vi "Fixed width File Parser.vi"(9 "Length of Column":i32[](array[numeric]), 10 "Start Index":i32[](array[numeric]), 11 "Folder to Check":path) -> (3 "Parsed Data":string[][](array[string]))   [LabVIEW 2009]
uses:
  <vilib>/Utility/file.llb/Read From Spreadsheet File (string).vi
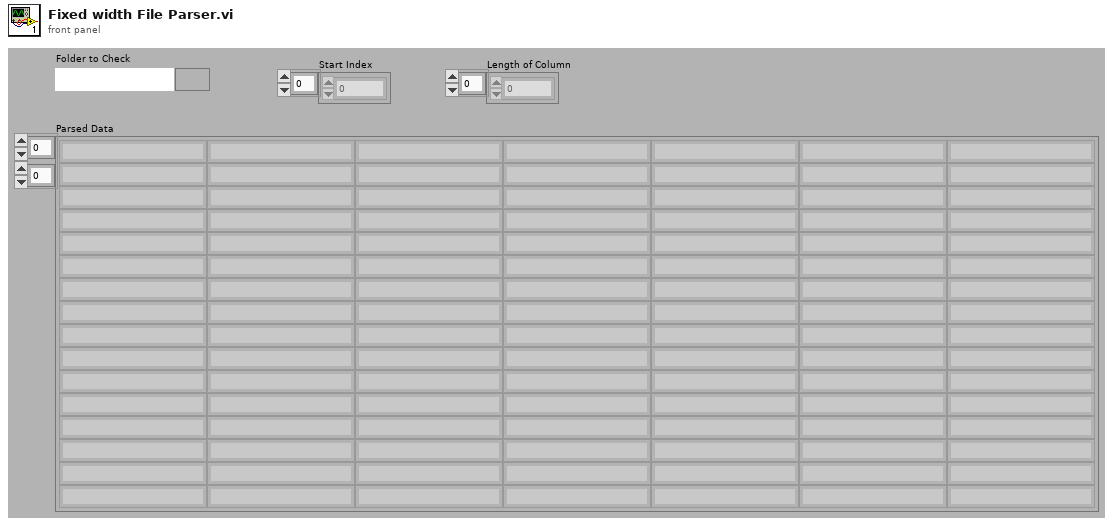
[diagram p1: front panel]
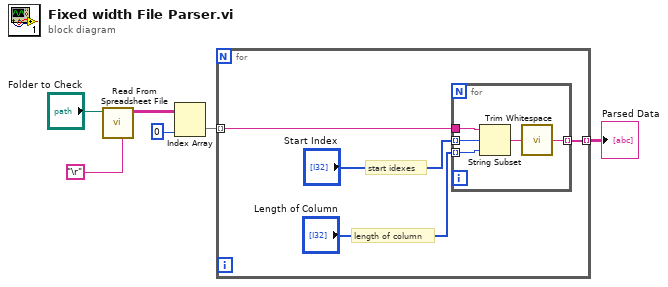
[diagram p0: block diagram]
diagram:
  n1 = call-poly <vilib>:"Read From Spreadsheet File.vi"("delimiter (\\t)"="\r", "file path (dialog if empty)"="Folder to Check") -> ("all rows"=w5:string[][])  [unwired: 5 in, 4 out]
  n2 = Index Array(array=w5, index (col)=0 ("disabled index (col)")) -> (element=w3:string[])  [unwired: 1 in]
  n3 = for {
    tunnel: w3 -> [w10] mode=indexing
    tunnel: [w9] -> w1 mode=indexing
    # "length of column"
    # "start idexes"
    n4 = for {
      tunnel: w10 -> [w13]
      tunnel: "Start Index" -> [w15] mode=indexing
      tunnel: "Length of Column" -> [w14] mode=indexing
      tunnel: [w11] -> w9 mode=indexing
      n5 = String Subset(string=w13, offset (0)=w15, length (rest)=w14) -> (substring=w12:string)
      n6 = call <vilib>:"Trim Whitespace.vi"("string"=w12) -> ("trimmed string"=w11:string)  [unwired: 1 in]
    }
  }
  "Parsed Data" <- w1
